vi "Render Missing Variable Key.vi"(8 "Error In":errorcluster) -> (0 "Error Out":errorcluster)   [LabVIEW 2018, in "Tests.lvlib" / "Render.lvlib"]
uses:
  Render.lvlib
  <vilib>/addons/_JKI Toolkits/Caraya/classes/Test/Test.lvclass
  <vilib>/addons/_JKI Toolkits/Caraya/classes/Assert/Assert.lvclass
  src/Toolkit/Toolkit.lvlib
  src/Toolkit/Low-Level/Support/Render to String.vi
  src/Toolkit/Data/Map/Map.lvclass
  src/Toolkit/Data/Map/Support/From String.vi
  src/Toolkit/Low-Level/Support/Lex String.vi
  src/Toolkit/Low-Level/Context/Compiler.lvclass
  D:/Users/cfield/Code/Field R&D Services/Labstache/src/Toolkit/Data/Datum/Datum.lvclass
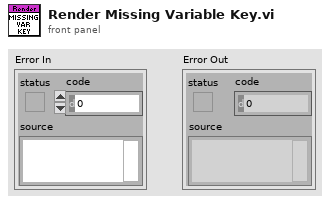
[diagram p1: front panel]
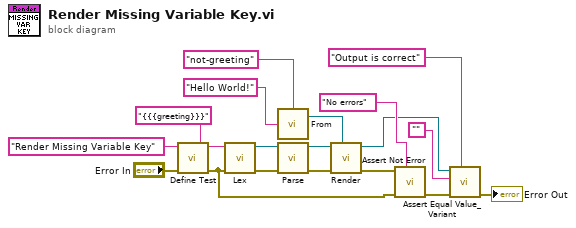
[diagram p0: block diagram]
diagram:
  n1 = call <vilib>:"Define Test.vi"("error in (no error)"="Error In", "Label (VI Title)"="Render Missing Variable Key") -> ("error out"=w2:errorcluster)  [unwired: 9 in]
  n2 = call-poly "Lex.vi"("Error In"=w2, "Context In"="{{{greeting}}}" ("format string")) -> ("Error Out"=w11:errorcluster, "Context Out"=w9:refnum<class "Compiler.lvclass">)  [unwired: 7 in, 1 out]
  n3 = call-poly "From.vi"("Value"="Hello World!", "Key"="not-greeting") -> ("Map"=w3:refnum<class "Map.lvclass">)
  n4 = call "Parse.vi"("Error In"=w11, "Context In"=w9) -> ("Error Out"=w8:errorcluster, "Context Out"=w7:refnum<class "Compiler.lvclass">)  [unwired: 7 in, 1 out]
  n5 = call-poly "Render.vi"(7:w3, "Error In"=w8, "Context In"=w7) -> ("Error Out"=w12:errorcluster, "Context Out"=w6:refnum<class "Compiler.lvclass">)  [unwired: 6 in, 1 out]
  n6 = call <vilib>:"Assert Not Error.vi"("Label"="No errors", "error in (no error)"=w2, "Not Error?"=w12) -> ("error out"=w15:errorcluster)  [unwired: 8 in]
  n7 = call <vilib>:"Assert Equal Value_Variant.vi"("Label"="Output is correct", "error in (no error)"=w15, "Y"="", "X"=w6) -> ("error out"=→"Error Out":errorcluster)  [unwired: 7 in]
